vi "runDOLT_img.vi"   [LabVIEW 2013]
types:
  T1 = cluster{"DOLT":refnum<k21>, "E_DOLT":errorcluster}
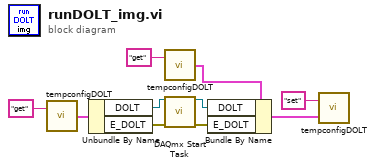
[diagram p0: block diagram]
diagram:
  n1 = call "tempconfigDOLT.vi"("command"="get") -> ("Temp Config out"=w9:T1)  [unwired: 1 in]
  n2 = Unbundle By Name(w9) -> ("DOLT"=w8:refnum<k21>, "E_DOLT"=w7:errorcluster)
  n3 = call "tempconfigDOLT.vi"("command"="get") -> ("Temp Config out"=w3:T1)  [unwired: 1 in]
  n4 = call <vilib>:"DAQmx Start Task.vi"("task/channels in"=w8, "error in"=w7) -> ("task out"=w6:refnum<k21>, "error out"=w5:errorcluster)  [unwired: 12 in]
  n5 = Bundle By Name(cluster=w3, "DOLT"=w6, "E_DOLT"=w5) -> (w1:T1)
  n6 = call "tempconfigDOLT.vi"("Temp Config in"=w1, "command"="set") -> ()  [unwired: 1 out]
